vi "Unregister Sensor Move In Next.vi"(8 "error in (no error)":errorcluster, 10 "View Enqueuer":refnum<class "Message Enqueuer.lvclass">, 11 "Sensor Model in":refnum<class "Sensor Model.lvclass">) -> (0 "error out":errorcluster, 3 "Sensor Model out":refnum<class "Sensor Model.lvclass">)   [LabVIEW 2013, in "Sensor Model.lvlib" / "Sensor Model.lvclass"]
uses:
  Sensor Model.lvclass
  <vilib>/ActorFramework/Message Enqueuer/Message Enqueuer.lvclass
  Sensor Model.lvclass/Sensor Model.ctl
  <vilib>/ActorFrameworkMVC/View Observer/View Registry/View Registry.lvclass
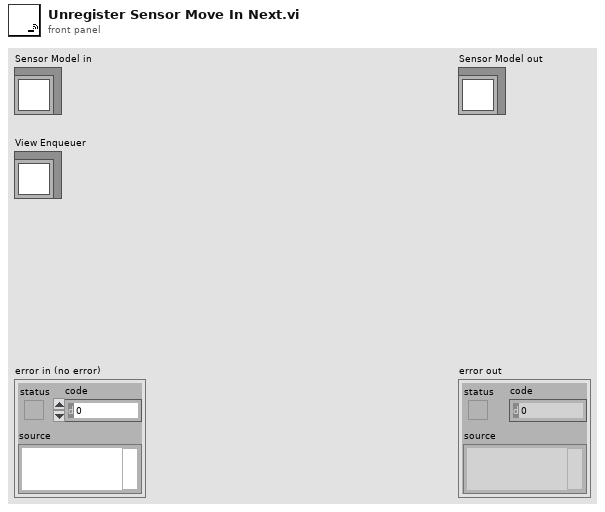
[diagram p1: front panel]
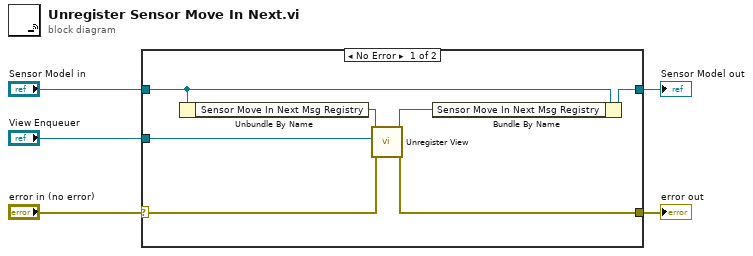
[diagram p0: block diagram]
diagram:
  n1 = case shown="No Error" "error in (no error)" {
    selector: "error in (no error)" -> [w10 w14]
    tunnel: "View Enqueuer" -> [w8 _]
    tunnel: "Sensor Model in" -> [w12 w13]
    tunnel: [w11 w13] -> w1
    tunnel: [w9 w14] -> w3
    frame No Error {
      n2 = Unbundle By Name(w12) -> ("Sensor Move In Next Msg Registry"=w7:refnum<class "View Registry.lvclass">)
      n3 = call <vilib>:"Unregister View.vi"("error in (no error)"=w10, "View Enqueuer"=w8, "View Registry in"=w7) -> ("error out"=w9:errorcluster, "View Registry out"=w6:refnum<class "View Registry.lvclass">)  [unwired: 7 in]
      n4 = Bundle By Name(cluster=w12, "Sensor Move In Next Msg Registry"=w6) -> (w11:refnum<class "Sensor Model.lvclass">)
    }
    frame Error {
    }
  }
  "error out" <- w3
  "Sensor Model out" <- w1
